vi "svl_Build Frame.vi"(2 "Y maximum":dbl format="%.2f", 3 "X maximum":dbl format="%.2f", 4 "z scale":cluster{"z min":dbl, "z max":dbl} {"z max" format="%.2f"; "z min" format="%.2f"}, 5 "x scale":cluster{"x min":dbl, "x max":dbl} {"x max" format="%.2f"; "x min" format="%.2f"}) -> (0 "back frame":cluster{dbl[], dbl[]} {"?" format="%.2f"; "?" format="%.2f"}, 1 "front frame":cluster{dbl[], dbl[]} {"?" format="%.2f"; "?" format="%.2f"})   [LabVIEW 2017]
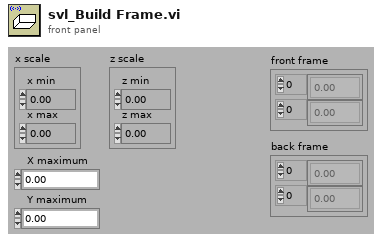
[diagram p1: front panel]
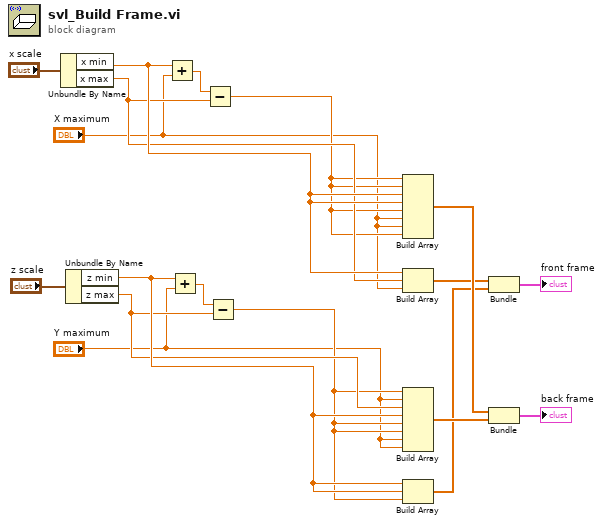
[diagram p0: block diagram]
diagram:
  n1 = Unbundle By Name("x scale") -> ("x min"=w9:dbl, "x max"=w8:dbl)
  n2 = Unbundle By Name("z scale") -> ("z min"=w6:dbl, "z max"=w5:dbl)
  n3 = Add(x=w9, y="X maximum") -> (x+y=w18:dbl)
  n4 = Add(x=w6, y="Y maximum") -> (x+y=w17:dbl)
  n5 = Subtract(x=w18, y=w8) -> (x-y=w4:dbl)
  n6 = Subtract(x=w17, y=w5) -> (x-y=w2:dbl)
  n7 = Build Array(w4, w4, w9, w9, w4, "X maximum", "X maximum", w4) -> (w16:dbl[])
  n8 = Build Array(w9, w8, "X maximum") -> (w13:dbl[])
  n9 = Build Array(w2, "Y maximum", w5, w6, w2, w2, "Y maximum", "Y maximum") -> (w15:dbl[])
  n10 = Build Array(w6, w6, w2) -> (w12:dbl[])
  n11 = Bundle(w13, w12) -> (→"front frame":cluster{dbl[], dbl[]})  [unwired: 1 in]
  n12 = Bundle(w16, w15) -> (→"back frame":cluster{dbl[], dbl[]})  [unwired: 1 in]
